vi "ex1_2.vi"() -> ()   [LabVIEW 2017]
uses:
  <vilib>/Analysis/2dsp.llb/Real FFT.vi
  <vilib>/Analysis/NI_AALPro.lvlib
panel:
  in  "stop":bool
  out "Max amplitude":dbl
  out "FFT for input 3":dbl[](graph)
  out "FFT for input 2":dbl[](graph)
  out "FFT for input 1":dbl[](graph)
  out "Y axis calibrated":dbl[](graph)
  out "Y axis normalized":dbl[](graph)
  out "FFT wihout mirror":dbl[](graph)
  out "Wave 3":dynamicdata(graph)
  out "Wave 2":dynamicdata(graph)
  out "Wave 1":dynamicdata(graph)
  out "FFT of superimposed signal (abs value)":dbl[](graph)
  out "Superimposed signal":dynamicdata(graph)
  in  "Select the status":bool
  in  "?":dbl
  in  "Frequency":dbl
  in  "Phase":dbl
  in  "?":dbl
  in  "Frequency":dbl
  in  "Phase":dbl
  in  "?":dbl
  in  "Frequency":dbl
  in  "Phase":dbl
  # "Amplitude"
  # "Amplitude"
  # "Amplitude"
  # "Not superimposed"
  # "Superimposed"
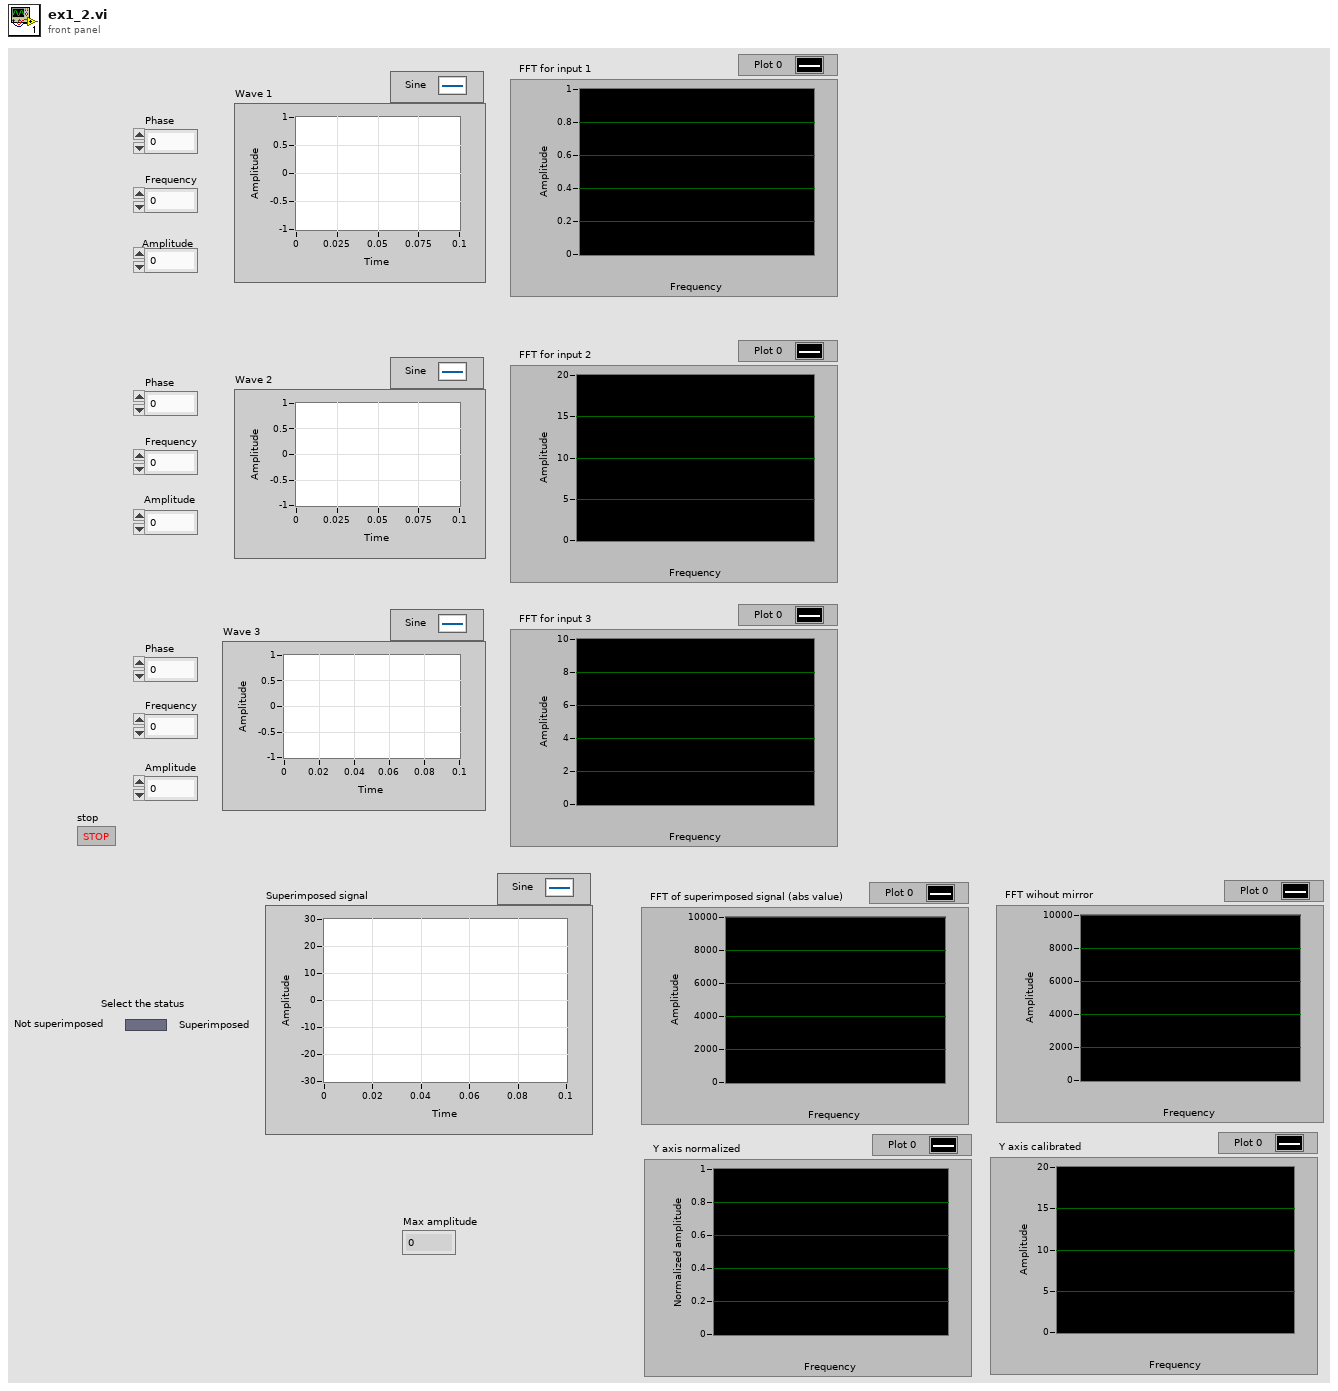
[diagram p1: front panel]
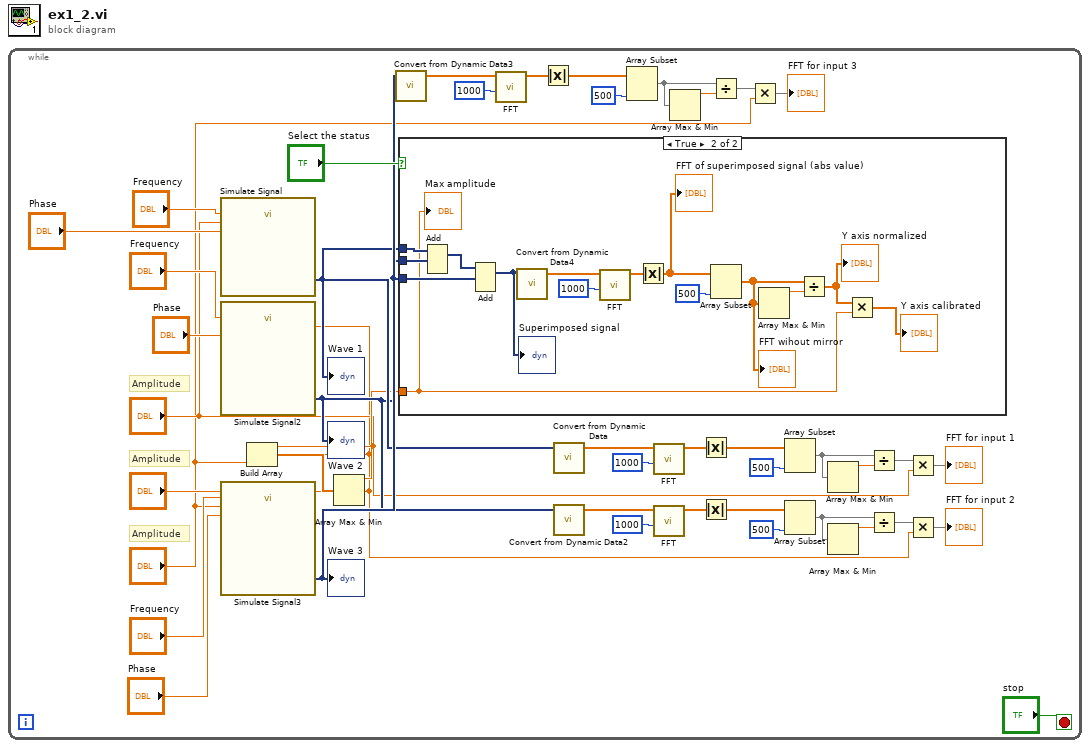
[diagram p0: block diagram]
diagram:
  n1 = while {
    stop <- "stop" stop-if-true
    # "Amplitude"
    # "Amplitude"
    # "Amplitude"
    n2 = call "Simulate Signal"("Frequency"="Frequency", "Amplitude"="?", "Phase"="Phase") -> ("Sine"=w29:dynamicdata)  [unwired: 11 in, 1 out]
    "Wave 1" <- w29
    n3 = call "Simulate Signal2"("Frequency"="Frequency", "Amplitude"="?", "Phase"="Phase") -> ("Sine"=w28:dynamicdata)  [unwired: 11 in, 1 out]
    "Wave 2" <- w28
    n4 = call "Simulate Signal3"("Frequency"="Frequency", "Amplitude"="?", "Phase"="Phase") -> ("Sine"=w30:dynamicdata)  [unwired: 11 in, 1 out]
    "Wave 3" <- w30
    n5 = Build Array("?", "?", "?") -> (w27:dbl[])
    n6 = Array Max & Min(array=w27) -> (max value=w26:dbl)  [unwired: 3 out]
    n7 = call "Convert from Dynamic Data3"("Dynamic Data Type"=w30) -> ("Array"=w32:dbl[])  [unwired: 3 in]
    n8 = case shown="True" "Select the status" {
      tunnel: w29 -> [_ w49]
      tunnel: w28 -> [_ w48]
      tunnel: w30 -> [_ w57]
      tunnel: w26 -> [_ w44]
      frame False {
      }
      frame True {
        n9 = Add(1:w48, 2:w49) -> (0:w58:dynamicdata)  [unwired: 1 in, 1 out]
        n10 = Add(1:w57, 2:w58) -> (0:w54:dynamicdata)  [unwired: 1 in, 1 out]
        "Superimposed signal" <- w54
        n11 = call "Convert from Dynamic Data4"("Dynamic Data Type"=w54) -> ("Array"=w56:dbl[])  [unwired: 3 in]
        n12 = call-poly <vilib>:"FFT.vi"("FFT size"=1000, "X"=w56) -> ("FFT {X}"=w53:cdb[])  [unwired: 8 in, 1 out]
        n13 = Absolute Value(x=w53) -> (abs(x)=w51:dbl[])
        "FFT of superimposed signal (abs value)" <- w51
        n14 = Array Subset(array=w51, length=500) -> (w45:dbl[])  [unwired: 1 in]
        "FFT wihout mirror" <- w45
        n15 = Array Max & Min(array=w45) -> (max value=w50:dbl)  [unwired: 3 out]
        n16 = Divide(x=w45, y=w50) -> (x/y=w47:dbl[])
        "Y axis normalized" <- w47
        n17 = Multiply(x=w47, y=w44) -> (x*y=→"Y axis calibrated":dbl[])
        "Max amplitude" <- w44
      }
    }
    n18 = call-poly <vilib>:"FFT.vi"("FFT size"=1000, "X"=w32) -> ("FFT {X}"=w4:cdb[])  [unwired: 8 in, 1 out]
    n19 = Absolute Value(x=w4) -> (abs(x)=w9:dbl[])
    n20 = call "Convert from Dynamic Data"("Dynamic Data Type"=w29) -> ("Array"=w36:dbl[])  [unwired: 3 in]
    n21 = call "Convert from Dynamic Data2"("Dynamic Data Type"=w28) -> ("Array"=w34:dbl[])  [unwired: 3 in]
    n22 = Array Subset(array=w9, length=500) -> (w6:dbl[])  [unwired: 1 in]
    n23 = call-poly <vilib>:"FFT.vi"("FFT size"=1000, "X"=w36) -> ("FFT {X}"=w23:cdb[])  [unwired: 8 in, 1 out]
    n24 = call-poly <vilib>:"FFT.vi"("FFT size"=1000, "X"=w34) -> ("FFT {X}"=w5:cdb[])  [unwired: 8 in, 1 out]
    n25 = Array Max & Min(array=w6) -> (max value=w10:dbl)  [unwired: 3 out]
    n26 = Absolute Value(x=w23) -> (abs(x)=w22:dbl[])
    n27 = Absolute Value(x=w5) -> (abs(x)=w15:dbl[])
    n28 = Divide(x=w6, y=w10) -> (x/y=w8:dbl[])
    n29 = Multiply(x=w8, y="?") -> (x*y=→"FFT for input 3":dbl[])
    n30 = Array Subset(array=w22, length=500) -> (w18:dbl[])  [unwired: 1 in]
    n31 = Array Subset(array=w15, length=500) -> (w12:dbl[])  [unwired: 1 in]
    n32 = Array Max & Min(array=w18) -> (max value=w24:dbl)  [unwired: 3 out]
    n33 = Array Max & Min(array=w12) -> (max value=w16:dbl)  [unwired: 3 out]
    n34 = Divide(x=w18, y=w24) -> (x/y=w21:dbl[])
    n35 = Divide(x=w12, y=w16) -> (x/y=w14:dbl[])
    n36 = Multiply(x=w21, y="?") -> (x*y=→"FFT for input 1":dbl[])
    n37 = Multiply(x=w14, y="?") -> (x*y=→"FFT for input 2":dbl[])
  }
